vi "Format Potting Config.vi"(8 "error in":errorcluster, 10 "Worktable":refnum<class "WorkTable Class.lvclass">, 11 "Console Log in":refnum<class "Console Log.lvclass">) -> (0 "error out":errorcluster, 2 "Formatted Worktable Config":string, 3 "Console Log out":refnum<class "Console Log.lvclass">)   [LabVIEW 2011, in "Console Log.lvclass"]
uses:
  Console Log.lvclass
  Shared Components/WorkTable Class/WorkTable Class.lvclass
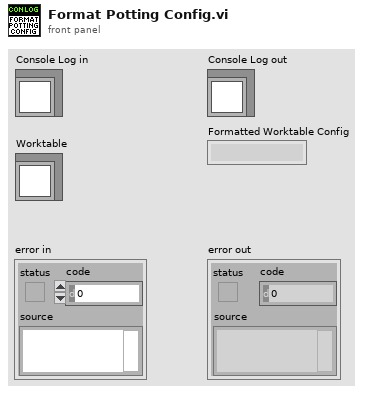
[diagram p1: front panel]
types:
  T1 = typedef "Worktable_Module Slot.ctl" = cluster{"Slot State":enum16{"Empty", "Bare HDI", "Unglued", "Stamped", "PartOnTop", "Weighted", "Unpotted", "Potted"}, "BBM Type":enum16{"None", "BBM", "GlassSlide"}, "HDI Type":enum16{"None", "HDI", "Polyimide"}, "Vacuum Channel":u8, "Location/Orientation BBM":T2, "Location/Orientation HDI":T2, "S/N":string}
  T2 = typedef "Position_Orientation.ctl" = cluster{"Center":refnum<class "Vec3d Class.lvclass">, "Orientation":refnum<class "Orient3d Class.lvclass">}
  T3 = enum16{"Empty", "Bare HDI", "Unglued", "Stamped", "PartOnTop", "Weighted", "Unpotted", "Potted"}
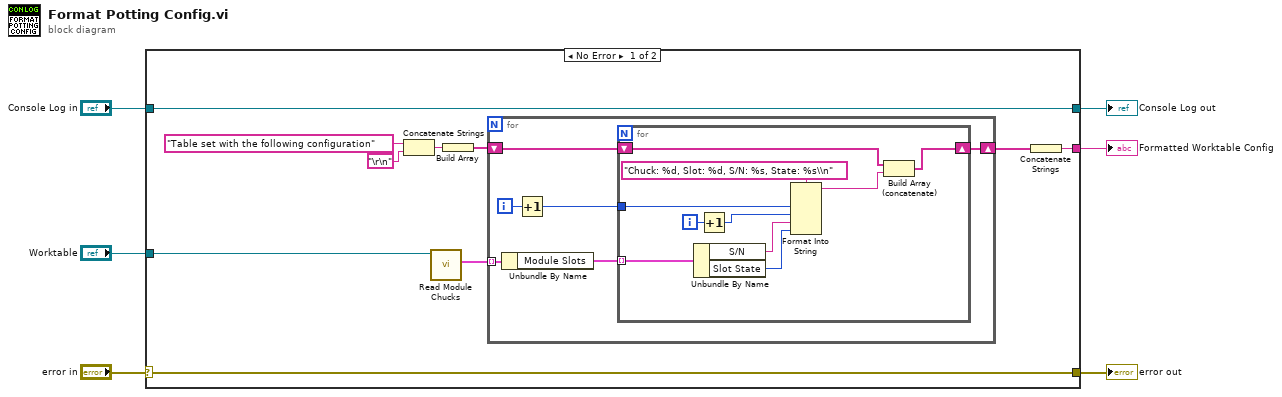
[diagram p0: block diagram]
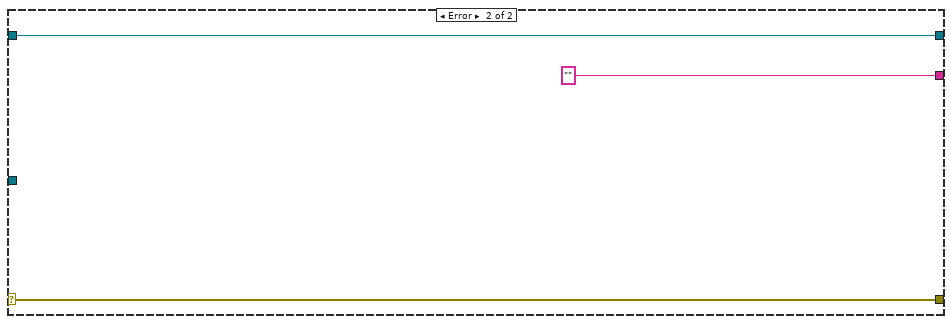
[diagram p2: hidden frame]
diagram:
  n1 = case shown="No Error" "error in" {
    selector: "error in" -> [w15 w35]
    tunnel: [w15 w35] -> w5
    tunnel: [w16 w34] -> w3
    tunnel: "Console Log in" -> [w16 w34]
    tunnel: "Worktable" -> [w14 _]
    tunnel: [w11 ""] -> w1
    frame No Error {
      n2 = Concatenate Strings("Table set with the following configuration", "\r\n") -> (w8:string)
      n3 = call-dynamic "Read Module Chucks.vi"("WorkTable in"=w14) -> ("Module Chucks"=w13:cluster{"Module Slots":T1[]}[])  [unwired: 8 in, 2 out]
      n4 = Build Array(w8) -> (w7:string[])
      n5 = for {
        tunnel: w13 -> [w22] mode=indexing
        shift-right: [w17] -> w12
        shift-left: w7 -> [w18]
        i -> [w20]
        n6 = Unbundle By Name(w22) -> ("Module Slots"=w21:T1[])
        n7 = Increment(x=w20) -> (x+1=w19:i32)
        n8 = for {
          tunnel: w21 -> [w32] mode=indexing
          tunnel: w19 -> [w30]
          shift-right: [w23] -> w17
          shift-left: w18 -> [w25]
          i -> [w31]
          n9 = Unbundle By Name(w32) -> ("S/N"=w27:string, "Slot State"=w26:T3)
          n10 = Increment(x=w31) -> (x+1=w29:i32)
          n11 = Format Into String(format string="Chuck: %d, Slot: %d, S/N: %s, State: %s\\n", w30, w29, w27, w26) -> (resulting string=w24:string)  [unwired: 2 in, 1 out]
          n12 = Build Array (concatenate)(w25, w24) -> (w23:string[])
        }
      }
      n13 = Concatenate Strings(w12) -> (w11:string)
    }
    frame Error {
    }
  }
  "error out" <- w5
  "Console Log out" <- w3
  "Formatted Worktable Config" <- w1
